vi "signal generator start.vi"(7 "source controls":T1={"signal choice"=FALSE, "amplitude"=1.0, "period"=50.0, "reset source"=FALSE} {"period" scale=1.0..1000.0; "amplitude" scale=0.0..2.0}) -> (8 "signal output":dbl)   [LabVIEW 2019]
doc: "this vi generates a sine or square wave point by point using a USR single shot\n\nPaul K Dixon\nP3600\nCSUSB Physics"
uses:
  typedefs/source control type.ctl
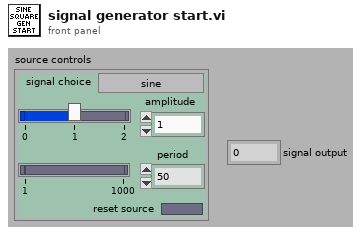
[diagram p1: front panel]
types:
  T1 = typedef "source control type.ctl" = cluster{"signal choice":bool, "amplitude":dbl, "period":dbl, "reset source":bool}
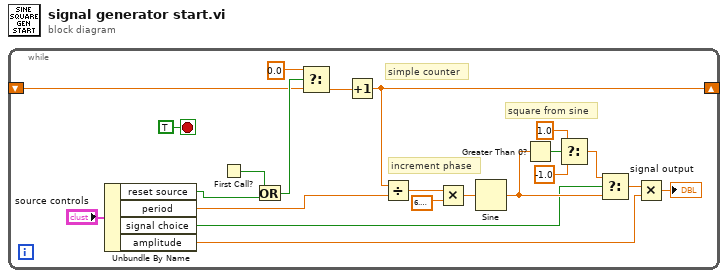
[diagram p0: block diagram]
diagram:
  n1 = while {
    shift-right: [w17] -> _
    shift-left: _ -> [w20]
    stop <- TRUE stop-if-true
    # "square from sine"
    # "increment phase"
    # "simple counter"
    n2 = Unbundle By Name("source controls") -> ("reset source"=w4:bool, "period"=w3:dbl, "signal choice"=w2:bool, "amplitude"=w1:dbl)
    n3 = First Call?() -> (First Call?: T/F=w9:bool)
    n4 = Or(x=w9, y=w4) -> (x .or. y?=w21:bool)
    n5 = Select(t=0.0, s=w21, f=w20) -> (s? t:f=w19:dbl)
    n6 = Increment(x=w19) -> (x+1=w17:dbl)
    n7 = Divide(x=w17, y=w3) -> (x/y=w14:dbl)
    n8 = Multiply(x=w14, y=6.283185307179586) -> (x*y=w13:dbl)
    n9 = Sine(x=w13) -> (sin(x)=w7:dbl)
    n10 = Greater Than 0?(x=w7) -> (x > 0?=w12:bool)
    n11 = Select(t=1.0, s=w12, f=-1.0) -> (s? t:f=w6:dbl)
    n12 = Select(t=w6, s=w2, f=w7) -> (s? t:f=w8:dbl)
    n13 = Multiply(x=w8, y=w1) -> (x*y=→"signal output":dbl)
  }
